vi "阈值处理图片.vi"() -> ()   [LabVIEW 2018]
uses:
  <vilib>/vision/NI_Vision_Development_Module.lvlib
panel:
  in  "退出标注":bool
  out "标注图":T1(plugin-control)
  out "阈值分割结果":T1(plugin-control)
  in  "Manual":cluster{sgl, sgl}(slide)={100.0, 255.0} caption="Threshold Range" scale=0.0..255.0
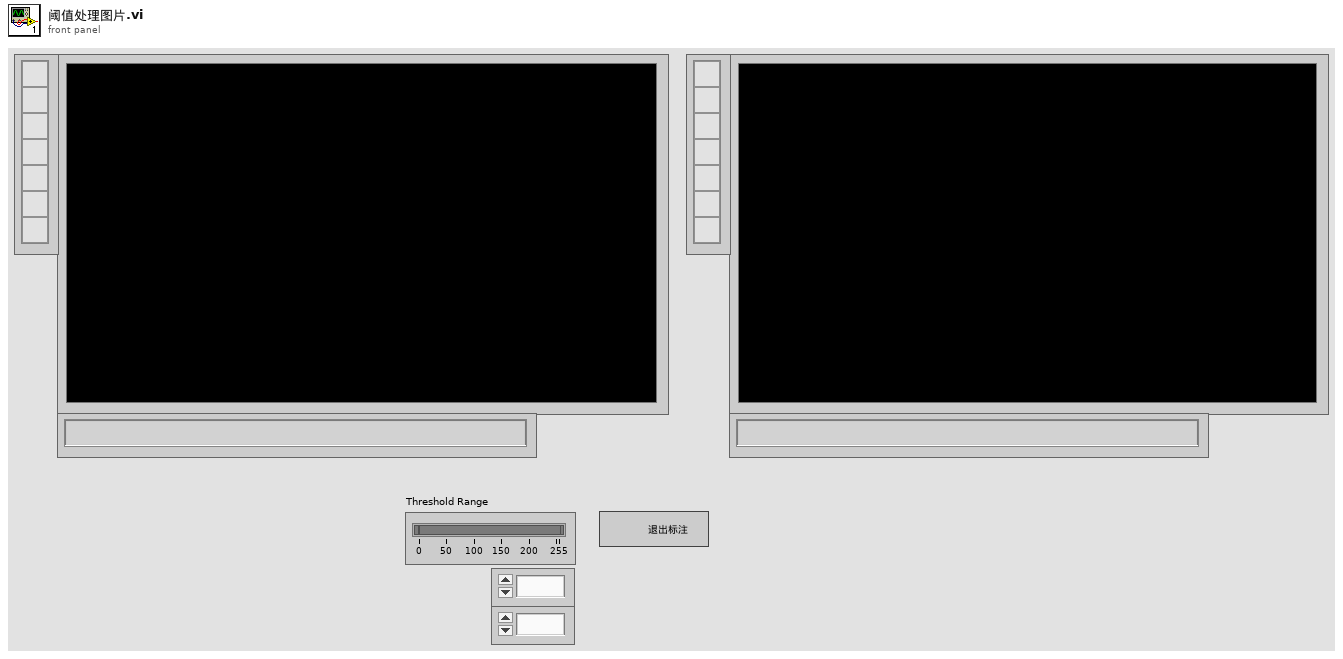
[diagram p1: front panel]
types:
  T1 = typedef "IMAQ Image.ctl" = refnum<image>
  T2 = typedef "Image Type" = u32
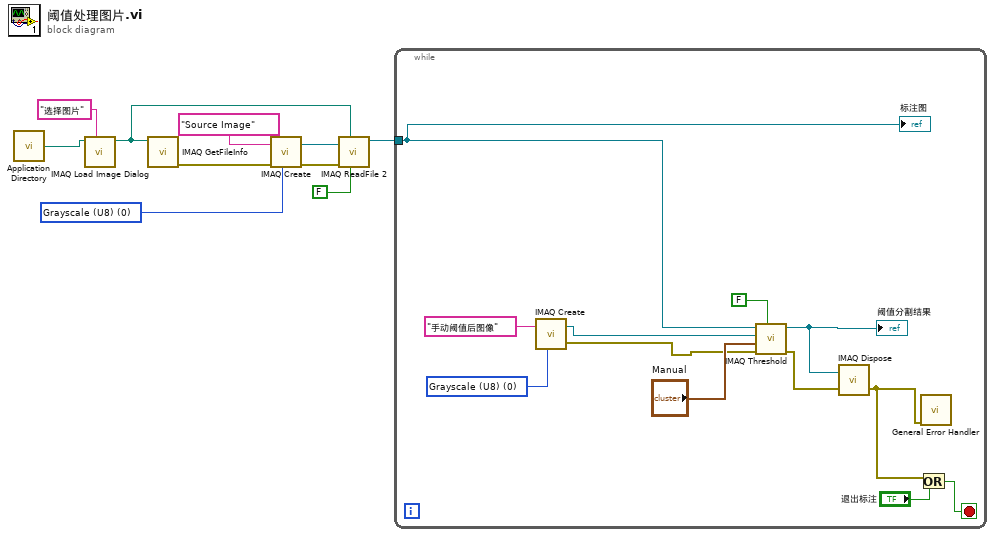
[diagram p0: block diagram]
diagram:
  w2 = T2 0 items=["Grayscale (U8)", "Grayscale (I16)", "Grayscale (SGL)", "Complex (CSG)", "RGB (U32)", "HSL (U32)", "RGB (U64)", "Grayscale (U16)"] ("Image Type")
  n1 = call <vilib>:"Application Directory.vi"() -> ("Application Directory"=w6:path)
  n2 = call "IMAQ Load Image Dialog"("Prompt"="选择图片" ("prompt"), "Start Path"=w6) -> ("Path"=w10:path)  [unwired: 7 in, 2 out]
  n3 = call "IMAQ GetFileInfo"("File Path"=w10) -> ("error out"=w9:errorcluster)  [unwired: 4 in, 6 out]
  n4 = call "IMAQ Create"("Image Name"="Source Image", "Image Type"=w2, "error in (no error)"=w9) -> ("New Image"=w8:T1, "error out"=w7:errorcluster)  [unwired: 2 in]
  n5 = call "IMAQ ReadFile 2"("Use File Path Image Type"=FALSE, "File Path"=w10, "error in (no error)"=w7, "Image"=w8) -> ("Image Out"=w1:T1)  [unwired: 3 in, 4 out]
  n6 = while {
    tunnel: w1 -> [w11]
    stop <- w13 stop-if-true
    w22 = T2 0 items=["Grayscale (U8)", "Grayscale (I16)", "Grayscale (SGL)", "Complex (CSG)", "RGB (U32)", "HSL (U32)", "RGB (U64)", "Grayscale (U16)"] ("Image Type")
    n7 = call "IMAQ Create"("Image Name"="手动阈值后图像", "Image Type"=w22) -> ("New Image"=w18:T1, "error out"=w17:errorcluster)  [unwired: 3 in]
    n8 = call "IMAQ Threshold"("Keep/Replace Value (Replace)"=FALSE, "error in (no error)"=w17, "Range"="Manual", "Image Dst"=w18, "Image Src"=w11) -> ("error out"=w15:errorcluster, "Image Dst Out"=w16:T1)  [unwired: 5 in]
    "阈值分割结果" <- w16
    n9 = call "IMAQ Dispose"("Image"=w16, "error in (no error)"=w15) -> ("error out"=w12:errorcluster)  [unwired: 1 in, 3 out]
    n10 = Or(x=w12, y="退出标注") -> (x .or. y?=w13:bool)
    n11 = call <vilib>:"General Error Handler.vi"("error in (no error)"=w12) -> ()  [unwired: 10 in, 5 out]
    "标注图" <- w11
  }
